vi "Configure Temperature.vi"(6 "Transducer Type":u16(ring) items=["Thermocouple", "Thermistor", "3-wire RTD", " 4-wire RTD"], 8 "error in (no error)":errorcluster, 9 "NPLC":u16(ring) items=["0.00005", "1", "12", "15"], 10 "Aperture Seconds":dbl, 11 "VISA resource name":refnum<visa-resource-name>) -> (0 "error out":errorcluster, 3 "VISA resource name out":refnum<visa-resource-name>)   [LabVIEW 2009, in "Keithley DMM7510.lvlib"]
doc: "This VI configures the Temperature measurement function parameters like transducer type, NPLC and the aperture setting."
uses:
  Keithley DMM7510.lvlib
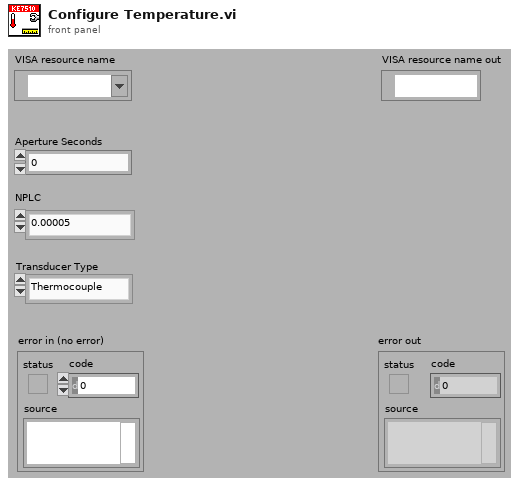
[diagram p1: front panel]
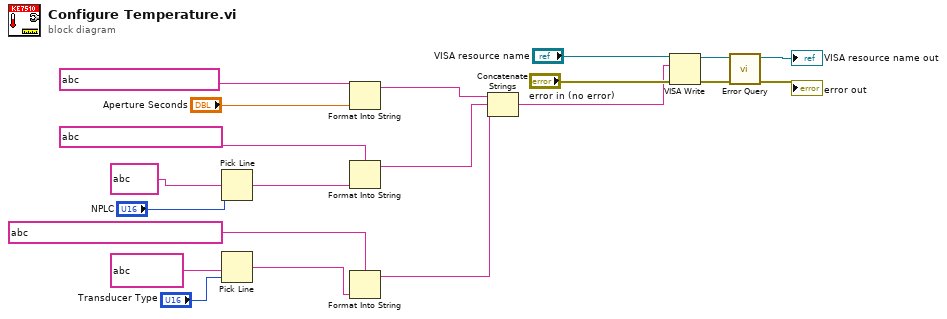
[diagram p0: block diagram]
diagram:
  n1 = Pick Line(multi-line string=string ?, line index="NPLC") -> (output string=w10:string)  [unwired: 1 in]
  n2 = Pick Line(multi-line string=string ?, line index="Transducer Type") -> (output string=w7:string)  [unwired: 1 in]
  n3 = Format Into String(format string=string ?, "Aperture Seconds") -> (resulting string=w15:string)  [unwired: 2 in, 1 out]
  n4 = Format Into String(format string=string ?, w10) -> (resulting string=w14:string)  [unwired: 2 in, 1 out]
  n5 = Format Into String(format string=string ?, w7) -> (resulting string=w5:string)  [unwired: 2 in, 1 out]
  n6 = Concatenate Strings(w15, w14, w5) -> (w13:string)
  n7 = VISA Write(VISA resource name="VISA resource name", write buffer=w13, error in (no error)="error in (no error)") -> (VISA resource name out=w4:refnum<visa-resource-name>, error out=w3:errorcluster)  [unwired: 1 out]
  n8 = call "Error Query.vi"("error in (no error)"=w3, "VISA resource name"=w4) -> ("error out"=→"error out":errorcluster, "VISA resource name out"=→"VISA resource name out":refnum<visa-resource-name>)  [unwired: 6 in, 2 out]
